vi "Register Clone with Framework.vi"(8 "error in (no error)":errorcluster, 11 "Application in":refnum<vi>) -> (0 "error out":errorcluster)   [LabVIEW 2022 SP3, in "Dummy.lvlib"]
doc: "\"Sets\" the module with the Framework (makes the UI Manager and Event Manager register for its broadcasts)\n\n____\nHAMPEL SOFTWARE ENGINEERING v2.6.0 (2023-12-19 10:54)"
uses:
  Dummy.lvlib
  Libraries/hse-libraries/Source/hse-application/hse-application.lvclass/hse-application.ctl
  Libraries/hse-libraries/Source/hse-application/HSE Application not initialized--error.vi
  <vilib>/Utility/error.llb/Clear Errors.vi
  Libraries/hse-libraries/Source/hse-application/hse-application__GetSingleton.vi
  <vilib>/Utility/sysdir.llb/Get System Directory.vi
  <vilib>/Utility/error.llb/Error Cluster From Error Code.vi
  Libraries/hse-libraries/Source/hse-dqmh/hse-dqmh-dynamicrequesters.lvlib
  Libraries/hse-libraries/Source/hse-application/hse-application.lvclass
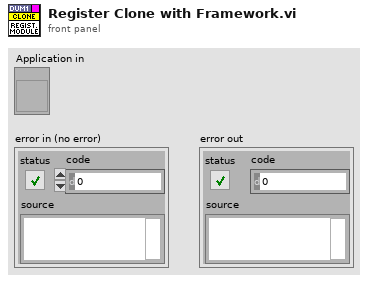
[diagram p1: front panel]
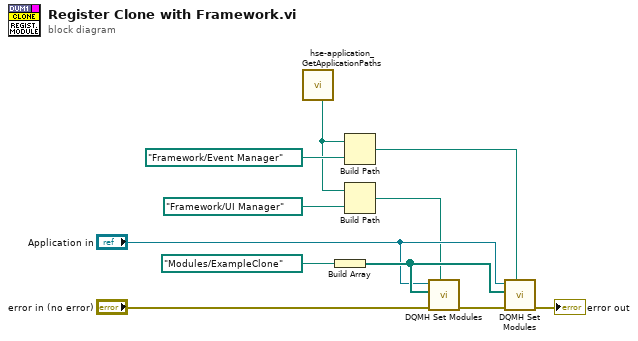
[diagram p0: block diagram]
diagram:
  n1 = call "hse-application_GetApplicationPaths.vi"() -> ("Application Base Path"=w8:path)  [unwired: 5 in, 6 out]
  n2 = Build Array(path "Modules/ExampleClone") -> (w7:path[])
  n3 = Build Path(base path=w8, name or relative path=path "Framework/Event Manager") -> (appended path=w10:path)
  n4 = Build Path(base path=w8, name or relative path=path "Framework/UI Manager") -> (appended path=w5:path)
  n5 = call "DQMH Set Modules.vi"("Module Disk Path"=w5, "error in (no error)"="error in (no error)", "modules to load dynamically"=w7, "Application reference"="Application in") -> ("error out"=w2:errorcluster)  [unwired: 7 in]
  n6 = call "DQMH Set Modules.vi"("Module Disk Path"=w10, "error in (no error)"=w2, "modules to load dynamically"=w7, "Application reference"="Application in") -> ("error out"=→"error out":errorcluster)  [unwired: 7 in]
